vi "MAIN - Acquire Data with Event.vi"() -> ()   [LabVIEW 2015]
uses:
  <vilib>/Platform/TimedLoop/XDataNode/timing_clust.ctl
  <vilib>/Platform/TimedLoop/XDataNode/nitl_modes.ctl
  <vilib>/Platform/TimedLoop/XDataNode/wakeup.ctl
  <vilib>/Platform/TimedLoop/XDataNode/XDataNode.xnode
  <vilib>/Platform/TimedLoop/XDataNode/XDNodeRunTimeDep.lvlib
panel:
  in  "event":bool
  out "Current Free Space (Mb)":dbl
  out "Low on Free Disk Space":bool
  in  "Save Type":u16(ring) items=["USB", "cRIO"]
  out "Buffer":dbl(slide) scale=0.0..1.0
  in  "Buffer Size":u32=1000
  out "timed out?":bool
  out "ticks in":u32
  out "Waveform Graph":dbl[][](graph)
  out "ticks out":u32
  out "Error":errorcluster
  in  "Record":bool
  in  "Filename":string="default.txt"
  in  "Stop":bool
  in  "Sampling Freq [Hz]":dbl=200.0
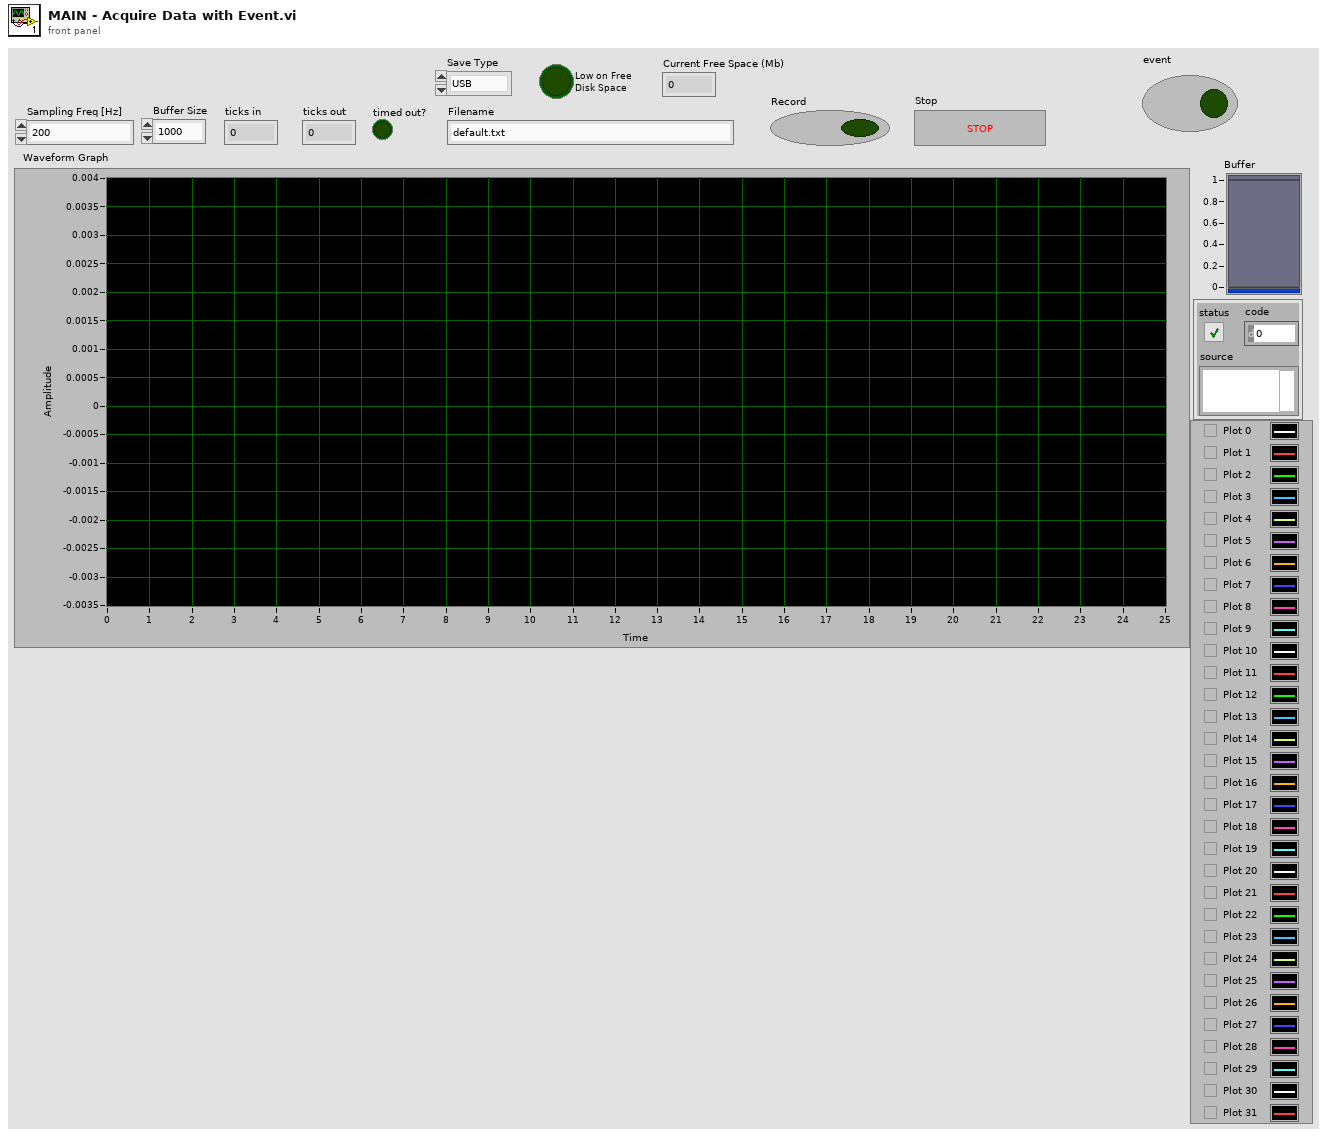
[diagram p1: front panel]
types:
  T1 = typedef "XDNodeRunTimeDep.lvlib/timing_clust.ctl" = cluster{"Expected End [f-1]":u64, "Actual End [f-1]":u64, "Finished Late? [f-1]":bool, "Expected End [i-1]":u64, "Actual End [i-1]":u64, "Finished Late? [i-1]":bool, "Expected Start [i]":u64, "Actual Start [i]":u64, "Expected Start [f]":u64, "Actual Start [f]":u64, "Source Name":string, "Structure Name":string, "Period":i64, "Deadline":i64, "Offset":i64, "Start":i64, "Priority":i32, "Timeout":i32, "Mode":T2, "Wakeup Reason":T3, "Error":errorcluster, "Source Type":string, "Secondary Source Type":string, "Global End Time":u64, "Global Start Time":u64, "Frame Duration":u64, "Iteration Duration":u64, "Assigned CPU":i32, "I/O Scan Engine Mode":u32}
  T2 = typedef "XDNodeRunTimeDep.lvlib/nitl_modes.ctl" = enum32{"No Change", "Process missed periods, maintain original phase", "Discard missed periods, maintain original phase", "Process missed periods, ignore original phase", "Discard missed periods, ignore original phase"}
  T3 = typedef "XDNodeRunTimeDep.lvlib/wakeup.ctl" = enum32{"Normal", "Aborted", "Asynchronous wakeup", "Timing source error", "Timed loop error", "Timeout"}
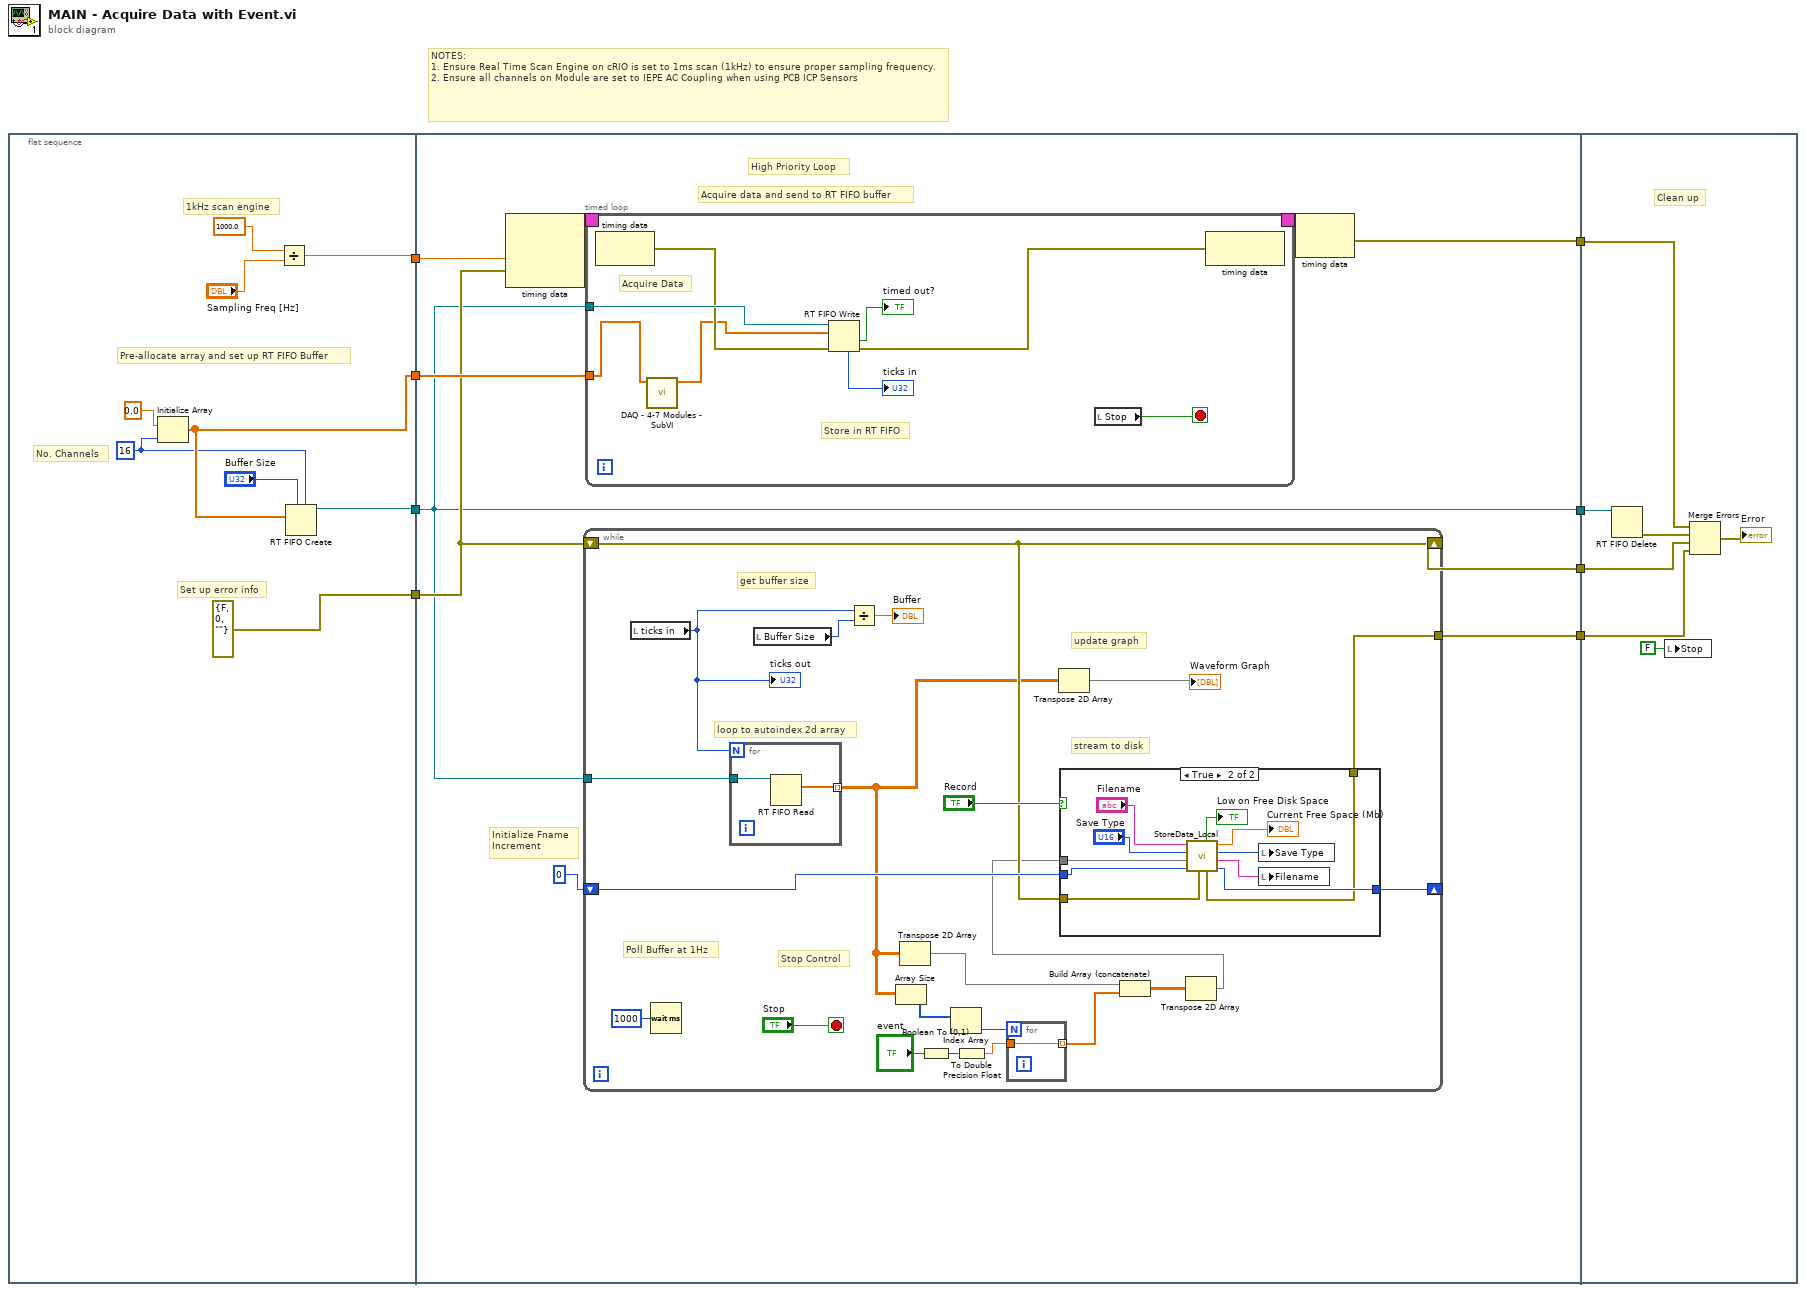
[diagram p0: block diagram]
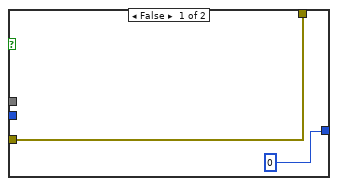
[diagram p2: hidden frame]
diagram:
  # "NOTES:\n1. Ensure Real Time Scan Engine on cRIO is set to 1ms scan (1kHz) to ensure proper sampling frequency.\n2. Ensure all channels on Module are set to IEPE AC Coupling when using PCB ICP Sensors"
  n1 = flat-sequence {
    tunnel: [w12] -> w8
    tunnel: [w17] -> w7
    tunnel: [w14] -> w6
    tunnel: [errorcluster {"status"=FALSE, "code"=0, "source"=""} ("Error")] -> w5
    tunnel: w8 -> [w25]
    tunnel: w7 -> [w24]
    tunnel: w6 -> [w20]
    tunnel: w5 -> [w23]
    tunnel: [w22] -> w4
    tunnel: [w21] -> w3
    tunnel: [w20] -> w2
    tunnel: [w19] -> w1
    tunnel: w4 -> [w91]
    tunnel: w3 -> [w86]
    tunnel: w2 -> [w88]
    tunnel: w1 -> [w85]
    frame #0 {
      w10 = 16 ("dimension size")
      # "No. Channels"
      # "Pre-allocate array and set up RT FIFO Buffer"
      # "1kHz scan engine"
      # "Set up error info"
      n2 = Initialize Array(0.0 ("element"), w10) -> (w12:dbl[])
      n3 = Divide(x=1000.0, y="Sampling Freq [Hz]") -> (x/y=w17:dbl)
      n4 = RT FIFO Create(1:w12, 4:"Buffer Size", 6:w10) -> (8:w14:refnum<k33>)  [unwired: 5 in, 2 out]
    }
    frame #1 {
      # "Initialize Fname \nIncrement"
      # "Acquire data and send to RT FIFO buffer"
      # "High Priority Loop"
      n5 = node-c288(w24, w23) -> (w27:T1)  [unwired: 1 in]
      n6 = while {
        tunnel: w20 -> [w48]
        shift-right: [w38] -> w21
        shift-left: w23 -> [w38]
        tunnel: [w41] -> w19
        shift-right: [w39] -> _
        shift-left: u8 0 -> [w40]
        stop <- "Stop" stop-if-true
        # "stream to disk"
        # "Stop Control"
        # "get buffer size"
        # "Poll Buffer at 1Hz"
        # "loop to autoindex 2d array"
        # "update graph"
        n7 = local read "ticks in"() -> (w43:u32)
        "ticks out" <- w43
        n8 = Wait (ms)(milliseconds to wait=u32 1000) -> ()  [unwired: 1 out]
        n9 = for {
          N: w43 -> [_]
          tunnel: [w52] -> w29 mode=indexing
          tunnel: w48 -> [w51]
          n10 = RT FIFO Read(0:w51) -> (9:w52:dbl[])  [unwired: 3 in, 4 out]
        }
        n11 = local read "Buffer Size"() -> (w42:u32)
        n12 = Divide(x=w43, y=w42) -> (x/y=→"Buffer":dbl)
        n13 = Array Size(array=w29) -> (size(s)=w35:i32[])
        n14 = Transpose 2D Array(2D array=w29) -> (transposed array=w31:dbl[][])
        n15 = Boolean To (0,1)(Boolean="event") -> (0, 1=w36:i16)
        n16 = Index Array(array=w35) -> (element=w34:i32)  [unwired: 1 in]
        n17 = To Double Precision Float(number=w36) -> (double precision float=w33:dbl)
        n18 = for {
          N: w34 -> [_]
          tunnel: w33 -> [w50]
          tunnel: [w50] -> w32 mode=indexing
        }
        n19 = Transpose 2D Array(2D array=w29) -> (transposed array=→"Waveform Graph":dbl[][])
        n20 = Build Array (concatenate)(w31, w32) -> (w30:dbl[][])
        n21 = Transpose 2D Array(2D array=w30) -> (transposed array=w28:dbl[][])
        n22 = case shown="True" "Record" {
          tunnel: w28 -> [_ w65]
          tunnel: [w53 w58] -> w41
          tunnel: w40 -> [_ w60]
          tunnel: [u8 0 w59] -> w39
          tunnel: w38 -> [w53 w55]
          frame False {
          }
          frame True {
            n23 = call "StoreData_Local.vi"("error in (no error)"=w55, "Fname Increment"=w60, "Array"=w65, "Save Type"="Save Type", "Filename"="Filename") -> ("NewFnameCount"=w59:u8, "New Fname"=w56:string, "New Save Type"=w57:u16, "Current Free Space (Mb)"=→"Current Free Space (Mb)":dbl, "error out"=w58:errorcluster, "Low on Free Disk Space"=→"Low on Free Disk Space":bool)  [unwired: 1 in]
            n24 = local write "Save Type"(w57) -> ()
            n25 = local write "Filename"(w56) -> ()
          }
        }
      }
      n26 = timed-loop {
        timing: w27 -> [_]
        timing-out: [_] -> w26
        tunnel: w25 -> [w67]
        tunnel: w20 -> [w73]
        stop <- w68 stop-if-true
        # "Store in RT FIFO"
        # "Acquire Data"
        n27 = node-c288() -> (w72:errorcluster)  [unwired: 1 in]
        n28 = call "DAQ - 4-7 Modules - SubVI.vi"("array"=w67) -> ("output array"=w66:dbl[])  [unwired: 10 in]
        n29 = RT FIFO Write(0:w73, 1:w66, 3:w72) -> (7:→"ticks in":u32, 10:→"timed out?":bool, 11:w71:errorcluster)  [unwired: 2 in, 1 out]
        n30 = local read "Stop"() -> (w68:bool)
        n31 = node-c288(w71) -> ()  [unwired: 1 out]
      }
      n32 = node-c288(w26) -> (w22:errorcluster)
    }
    frame #2 {
      # "Clean up"
      n33 = RT FIFO Delete(0:w88) -> (11:w87:errorcluster)  [unwired: 2 in]
      n34 = local write "Stop"(FALSE ("Stop")) -> ()
      n35 = Merge Errors(w91, w87, w86, w85) -> (→"Error":errorcluster)
    }
  }
